vi "PH_Timing.set Attr and open DIM Services.vi"(0 "i ref in":refnum<vi>, 5 "error in (no error)":errorcluster) -> (14 "i ref out":refnum<vi>, 16 "i Attr":T1={"Sequencer"={"linked?"=FALSE, "Proc State"="no info", "Ref State"=refnum}, "Gate Generator"={"GD"={"Device Status"=0, "linked?"=FALSE}, "Settings"={"Instance"="N/A", "Channel Gate"=1, "Channel T2"=1, "Width Gate"=1.0, "Width T2"=1.0, "Delay Gate"=0.0, "Delay T2"=0.0, "Gate activ"=FALSE, "T2 activ"=FALSE, "System Mode"=enum."Normal"}, "GUI Ref"=refnum}, "Interlock Bypass"={"Instancename"="N/A", "Switch linked?"=FALSE, "Device Status"=0, "Ref Status"=refnum}, "Roughtuner"={"Settings"={"Instance"="N/A", "Phase PHELIX / UNILAC"={"Channel"=0, "relative to"=0, "Delay [ms]"=0.0}, "Pulse Length"={"Channel"=0, "relative to"=0, "Delay [ms]"=0.0}, "Trigger"={"externally?"=FALSE, "Rate [Hz]"=0.0}}, "GUI Ref"=refnum, "GD"={"Device Status"=0, "linked?"=FALSE}}, "0,5Hz Gater"={"Settings"={"Instance"="N/A", "Channel ns FE Delay"=1, "Channel 0.5Hz"=1, "Width ns FE Delay"=1.0, "Width 0.5Hz"=1.0, "Delay ns FE Delay"=0.0, "Delay 0.5Hz"=0.0, "ns FE Delay active"=FALSE, "0.5Hz activ"=FALSE, "ns FE Delay inverted"=FALSE, "0.5Hz inverted"=FALSE}, "GUI Ref"=refnum, "GD"={"Device Status"=0, "linked?"=FALSE}}, "Slow Trigger"={"Settings"={"Delay"=0.0, "externally triggered?"=FALSE}, "GUI Ref"=refnum, "Service ID Delay"=-1, "Service ID Ext Trig"=-1, "Wanted Settings"={"Delay"=0.0, "externally triggered?"=FALSE}}, "Timing Mode"={"Mode"={"T2"=0, "Modeselector"=enum."0.5 Hz"}, "GUI Ref"=refnum, "Service ID T2"=-1, "Service ID Mode"=-1, "Wanted Mode"={"T2"=0, "Modeselector"=enum."10 Hz"}}, "ns Generator"={"Settings"={"Instance"="N/A", "Phase fs / ns FE"={"Channel"=0, "Settings"={"Delay [s]"=0.0, "relative to"=0}}}, "ns Generator Settings"=refnum, "GD"={"Device Status"=0, "linked?"=FALSE}}, "Phase FEs"={"Settings"={"Phase"=0.0}, "GUI Ref"=refnum, "Service ID Phase"=-1, "Wanted Settings"={"Phase"=0.0}}, "GD GUI Refs"=[], "Heads"=[], "GUI Ref Delete"=refnum} {"Heads"."GD"."Device Status" items=["no info", "off/false/out", "on/true/in", "Failure", "Alarm", "Status 1", "Status 2", "Status 3"]; "Heads"."Data"."CH" items=["System (To)", "Channel A", "Channel B", "Channel C", "Channel D", "Channel E", "Channel F", "Channel G", "Channel H"]; "Heads"."Data"."Delay" format="%#_7f"; "Phase FEs"."Wanted Settings"."Phase" format="%#_12p"; "Phase FEs"."Settings"."Phase" format="%#_12p"; "ns Generator"."GD"."Device Status" items=["no info", "off/false/out", "on/true/in", "Failure", "Alarm", "Status 1", "Status 2", "Status 3"]; "ns Generator"."Settings"."Phase fs / ns FE"."Settings"."relative to" items=["T0", "T1", "A", "B", "C", "D", "E", "F", "G", "H"]; "ns Generator"."Settings"."Phase fs / ns FE"."Settings"."Delay [s]" format="%#_12p"; "ns Generator"."Settings"."Phase fs / ns FE"."Channel" items=["T0", "T1", "A", "B", "C", "D", "E", "F", "G", "H"]; "Timing Mode"."Wanted Mode"."T2" min=0 max=6000 step=2; "Timing Mode"."Mode"."T2" min=0 max=6000 step=2; "0,5Hz Gater"."GD"."Device Status" items=["no info", "off/false/out", "on/true/in", "Failure", "Alarm", "Status 1", "Status 2", "Status 3"]; "0,5Hz Gater"."Settings"."Channel ns FE Delay" items=["System (To)", "Channel A", "Channel B", "Channel C", "Channel D", "Channel E", "Channel F", "Channel G", "Channel H"]; "0,5Hz Gater"."Settings"."Channel 0.5Hz" items=["System (To)", "Channel A", "Channel B", "Channel C", "Channel D", "Channel E", "Channel F", "Channel G", "Channel H"]; "Roughtuner"."GD"."Device Status" items=["no info", "off/false/out", "on/true/in", "Failure", "Alarm", "Status 1", "Status 2", "Status 3"]; "Roughtuner"."Settings"."Pulse Length"."Delay [ms]" format="%#_8g"; "Roughtuner"."Settings"."Pulse Length"."relative to" items=["T0", "A", "B", "AB", "C", "D", "CD"]; "Roughtuner"."Settings"."Pulse Length"."Channel" items=["T0", "A", "B", "AB", "C", "D", "CD"]; "Roughtuner"."Settings"."Phase PHELIX / UNILAC"."Delay [ms]" format="%#_8g"; "Roughtuner"."Settings"."Phase PHELIX / UNILAC"."relative to" items=["T0", "A", "B", "AB", "C", "D", "CD"]; "Roughtuner"."Settings"."Phase PHELIX / UNILAC"."Channel" items=["T0", "A", "B", "AB", "C", "D", "CD"]; "Interlock Bypass"."Device Status" items=["no info", "off/false/out", "on/true/in", "Failure", "Alarm", "Status 1", "Status 2", "Status 3"]; "Gate Generator"."Settings"."Channel Gate" items=["System (To)", "Channel A", "Channel B", "Channel C", "Channel D", "Channel E", "Channel F", "Channel G", "Channel H"]; "Gate Generator"."Settings"."Channel T2" items=["System (To)", "Channel A", "Channel B", "Channel C", "Channel D", "Channel E", "Channel F", "Channel G", "Channel H"]; "Gate Generator"."GD"."Device Status" items=["no info", "off/false/out", "on/true/in", "Failure", "Alarm", "Status 1", "Status 2", "Status 3"]}, 19 "error out":errorcluster)   [LabVIEW 2014, in "PH_Timing.lvlib"]
doc: "In this VI the related instances which are not set in the Read DB Vi are defined and set (includinbg default values) to own attributes."
uses:
  PH_Timing.lvlib
  PH_Timing.i attribute.ctl
  PH_Basics/PH_StatusHandler/PH_StatusHandler.Status.ctl
  PH_Timing.GateGen.ctl
  PH_Timing.Roughtuner.ctl
  PH_Timing.0.5HzGater.ctl
  PH_Timing.Slow Trigger Settings.ctl
  PH_Timing.Timing Mode.ctl
  PH_Timing.ns Generator.ctl
  instr.lib/SRDG645/Driver/Channel.ctl
  PH_Devices/PH_SRDG645/PH_SRDG645.Channel Settings.ctl
  PH_Timing.Phase FEs.ctl
  PH_Timing.PU Data.ctl
  PH_Timing.PU Info.ctl
  PH_Basics/PH_PP_Common/PH_PP_Common.PUs.ctl
  CS_DigitalIO/SRDG535/SRDG535.Channel.ctl
  CS_DigitalIO/SRDG535/SRDG535.lvlib
  instr.lib/SRDG645/Stanford Research DG645 - Driver.lvlib
  PH_Basics/PH_StatusHandler/PH_StatusHandler.lvlib
  PH_Devices/PH_SRDG645/PH_SRDG645.lvlib
  PH_Basics/PH_Common/PH_Common.lvlib
  PH_Basics/PH_PP_Common/PH_PP_Common.lvlib
  CS_Core/CSSystem/CSSystemLib/CSSystemLib.lvlib
panel:
  # "s"
  # "s"
  # "AND ns FE Delay"
  # "AND 0.5 Hz"
  # "Gate"
  # "T2"
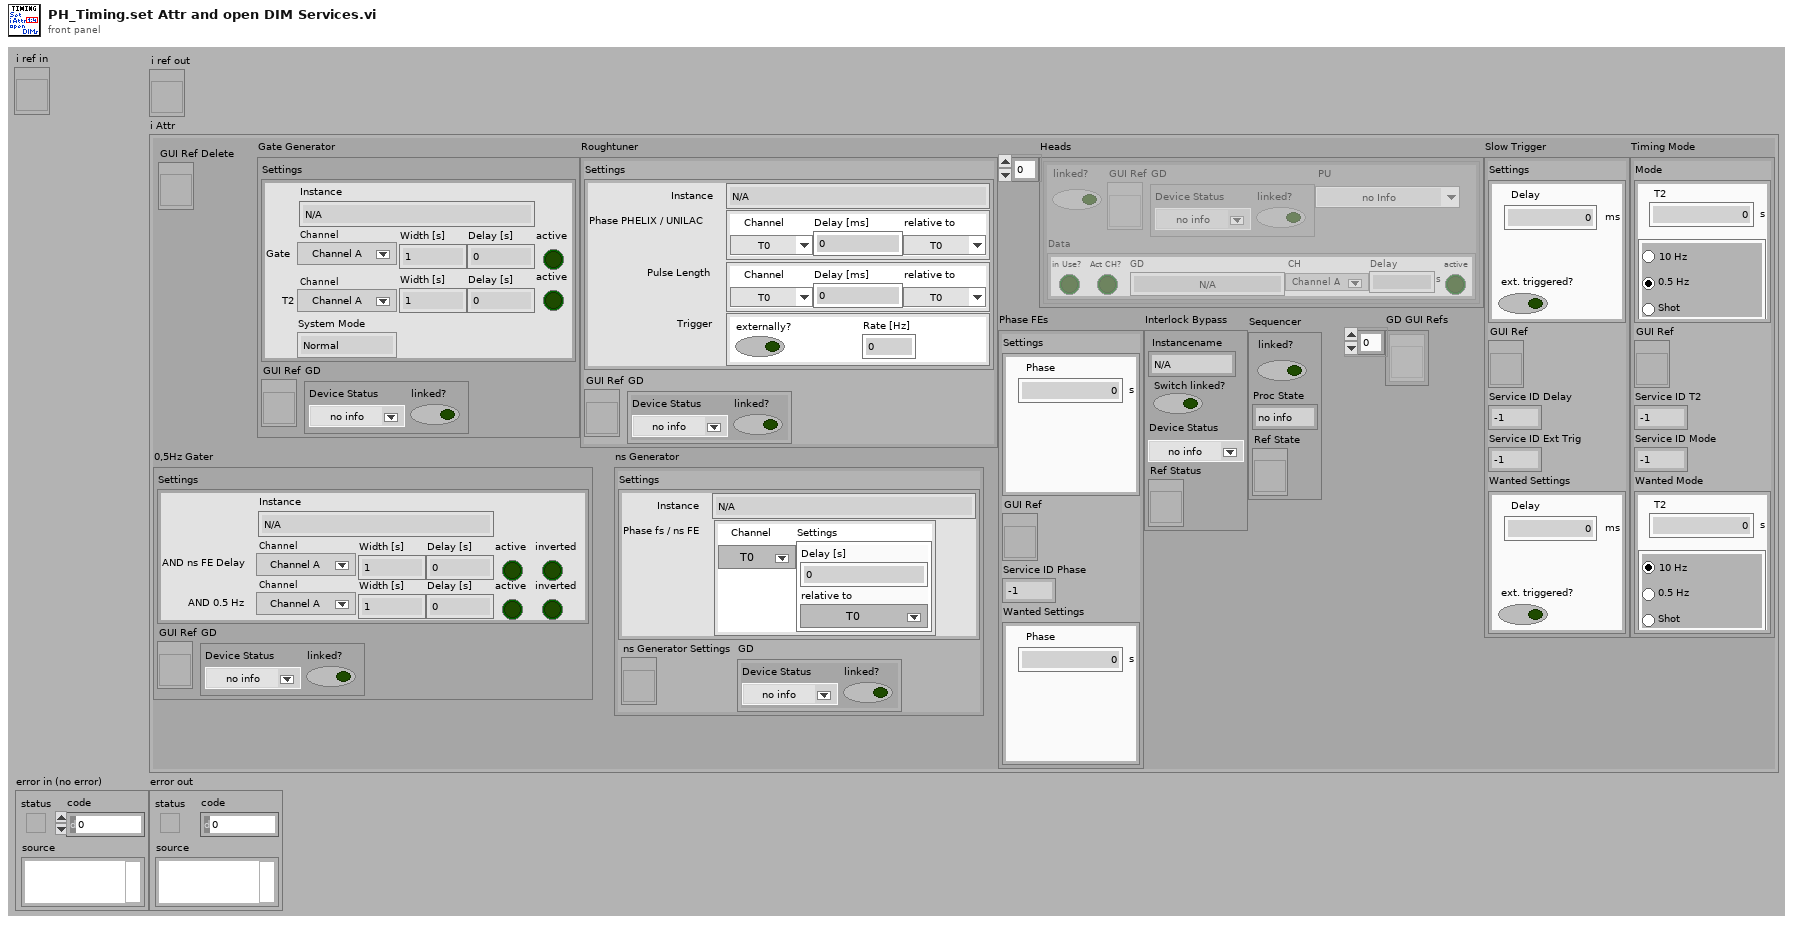
[diagram p1: front panel]
types:
  T1 = typedef "PH_Timing.lvlib/PH_Timing.i attribute.ctl" = cluster{"Sequencer":cluster{"linked?":bool, "Proc State":string, "Ref State":refnum<vi>}, "Gate Generator":cluster{"GD":cluster{"Device Status":T2, "linked?":bool}, "Settings":T3, "GUI Ref":refnum<vi>}, "Interlock Bypass":cluster{"Instancename":string, "Switch linked?":bool, "Device Status":T2, "Ref Status":refnum<vi>}, "Roughtuner":cluster{"Settings":T4, "GUI Ref":refnum<vi>, "GD":cluster{"Device Status":T2, "linked?":bool}}, "0,5Hz Gater":cluster{"Settings":T5, "GUI Ref":refnum<vi>, "GD":cluster{"Device Status":T2, "linked?":bool}}, "Slow Trigger":cluster{"Settings":T6, "GUI Ref":refnum<vi>, "Service ID Delay":i32, "Service ID Ext Trig":i32, "Wanted Settings":T6}, "Timing Mode":cluster{"Mode":T7, "GUI Ref":refnum<vi>, "Service ID T2":i32, "Service ID Mode":i32, "Wanted Mode":T7}, "ns Generator":cluster{"Settings":T8, "ns Generator Settings":refnum<vi>, "GD":cluster{"Device Status":T2, "linked?":bool}}, "Phase FEs":cluster{"Settings":T11, "GUI Ref":refnum<vi>, "Service ID Phase":i32, "Wanted Settings":T11}, "GD GUI Refs":refnum<vi>[], "Heads":T12[], "GUI Ref Delete":refnum<vi>}
  T2 = typedef "PH_StatusHandler.lvlib/PH_StatusHandler.Status.ctl" = i16
  T3 = typedef "PH_Timing.lvlib/PH_Timing.GateGen.ctl" = cluster{"Instance":string, "Channel Gate":i32, "Channel T2":i32, "Width Gate":dbl, "Width T2":dbl, "Delay Gate":dbl, "Delay T2":dbl, "Gate activ":bool, "T2 activ":bool, "System Mode":enum16{"Normal", "Single", "Burst", "Duty Cycle"}}
  T4 = typedef "PH_Timing.lvlib/PH_Timing.Roughtuner.ctl" = cluster{"Instance":string, "Phase PHELIX / UNILAC":cluster{"Channel":u16, "relative to":u16, "Delay [ms]":dbl}, "Pulse Length":cluster{"Channel":u16, "relative to":u16, "Delay [ms]":dbl}, "Trigger":cluster{"externally?":bool, "Rate [Hz]":dbl}}
  T5 = typedef "PH_Timing.lvlib/PH_Timing.0.5HzGater.ctl" = cluster{"Instance":string, "Channel ns FE Delay":i32, "Channel 0.5Hz":i32, "Width ns FE Delay":dbl, "Width 0.5Hz":dbl, "Delay ns FE Delay":dbl, "Delay 0.5Hz":dbl, "ns FE Delay active":bool, "0.5Hz activ":bool, "ns FE Delay inverted":bool, "0.5Hz inverted":bool}
  T6 = typedef "PH_Timing.lvlib/PH_Timing.Slow Trigger Settings.ctl" = cluster{"Delay":dbl, "externally triggered?":bool}
  T7 = typedef "PH_Timing.lvlib/PH_Timing.Timing Mode.ctl" = cluster{"T2":i16, "Modeselector":enum32{"10 Hz", "0.5 Hz", "Shot"}}
  T8 = typedef "PH_Timing.lvlib/PH_Timing.ns Generator.ctl" = cluster{"Instance":string, "Phase fs / ns FE":cluster{"Channel":T9, "Settings":T10}}
  T9 = typedef "Stanford Research DG645 - Driver.lvlib/Channel.ctl" = i32
  T10 = typedef "PH_SRDG645.lvlib/PH_SRDG645.Channel Settings.ctl" = cluster{"Delay [s]":dbl, "relative to":i32}
  T11 = typedef "PH_Timing.lvlib/PH_Timing.Phase FEs.ctl" = cluster{"Phase":dbl}
  T12 = typedef "PH_Timing.lvlib/PH_Timing.PU Data.ctl" = cluster{"linked?":bool, "Data":T13, "GD":cluster{"Device Status":T2, "linked?":bool}, "GUI Ref":refnum<vi>, "PU":T14}
  T13 = typedef "PH_Timing.lvlib/PH_Timing.PU Info.ctl" = cluster{"Act CH?":bool, "GD":string, "CH":i32, "Delay":dbl, "active":bool, "in Use?":bool}
  T14 = typedef "PH_PP_Common.lvlib/PH_PP_Common.PUs.ctl" = enum16{"no Info", "PA-19mm-1", "PA-19mm-2", "PA-45mm-PILC", "PA-45mm-MAIN", "MA-PU-1", "MA-PU-2", "MA-PU-3", "MA-PU-4", "MA-PU-5", "MA-PU-6", "MA-FR", "MA-PILC", "PA-45mm-DP"}
  T15 = typedef "SRDG535.lvlib/SRDG535.Channel.ctl" = u16
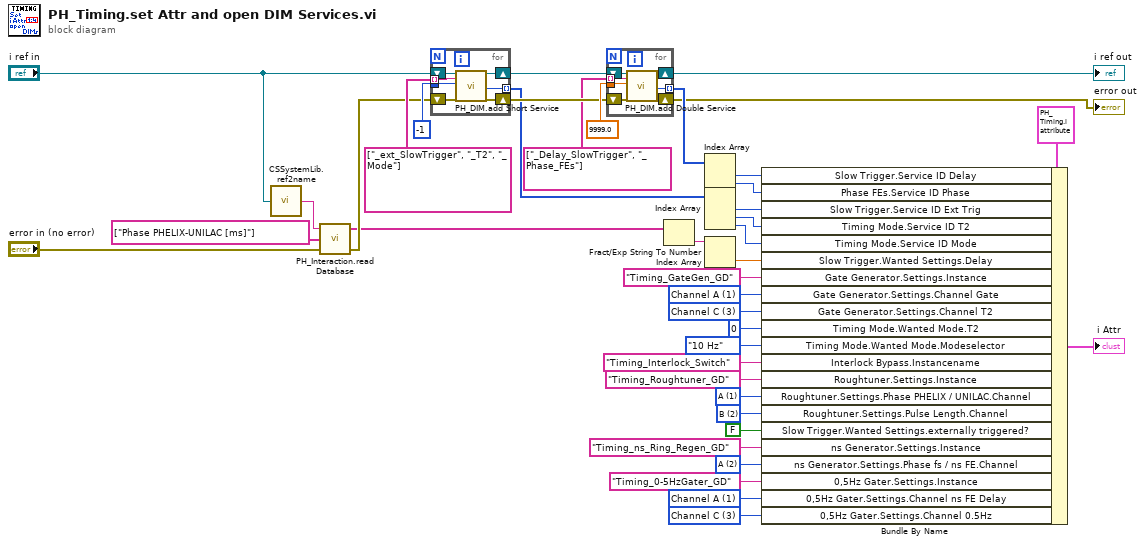
[diagram p0: block diagram]
diagram:
  w15 = T9 2 items=["T0", "T1", "A", "B", "C", "D", "E", "F", "G", "H"] ("ns Generator.Settings.Phase fs / ns FE.Channel")
  w34 = T15 2 items=["T0", "A", "B", "AB", "C", "D", "CD"] ("Channel")
  w35 = T15 1 items=["T0", "A", "B", "AB", "C", "D", "CD"] ("Channel")
  w37 = 3 items=["System (To)", "Channel A", "Channel B", "Channel C", "Channel D", "Channel E", "Channel F", "Channel G", "Channel H"] ("Channel Gate T0")
  w38 = 1 items=["System (To)", "Channel A", "Channel B", "Channel C", "Channel D", "Channel E", "Channel F", "Channel G", "Channel H"] ("Channel Gate T0")
  w39 = 3 items=["System (To)", "Channel A", "Channel B", "Channel C", "Channel D", "Channel E", "Channel F", "Channel G", "Channel H"] ("Channel Gate T0")
  w40 = 1 items=["System (To)", "Channel A", "Channel B", "Channel C", "Channel D", "Channel E", "Channel F", "Channel G", "Channel H"] ("Channel Gate T0")
  n1 = call "CSSystemLib.ref2name.vi"("obj refnum"="i ref in") -> ("name"=w11:string)
  n2 = call "PH_Interaction.read Database.vi"("error in (no error)"="error in (no error)", "Strings to search for"=string[] ["Phase PHELIX-UNILAC [ms]"], "DB Entry to read"=w11) -> ("error out"=w13:errorcluster, "Values"=w12:string[])  [unwired: 1 in]
  n3 = for {
    tunnel: i16 -1 ("Number") -> [w45]
    shift-right: [w47] -> w27
    shift-left: "i ref in" -> [w44]
    shift-right: [w46] -> w26
    shift-left: w13 -> [w43]
    tunnel: string[] ["_ext_SlowTrigger", "_T2", "_Mode"] -> [w42] mode=indexing
    tunnel: [w41] -> w23 mode=indexing
    n4 = call "PH_DIM.add Short Service.vi"("i ref in"=w44, "Service Name"=w42, "Number"=w45, "error in (no error)"=w43) -> ("i ref out"=w47:refnum<vi>, "Service ID"=w41:i32, "error out"=w46:errorcluster)  [unwired: 13 in]
  }
  n5 = for {
    tunnel: 9999.0 ("Double Value") -> [w52]
    tunnel: [w49] -> w21 mode=indexing
    tunnel: string[] ["_Delay_SlowTrigger", "_Phase_FEs"] -> [w48] mode=indexing
    shift-right: [w54] -> w2
    shift-left: w27 -> [w51]
    shift-right: [w53] -> w1
    shift-left: w26 -> [w50]
    n6 = call "PH_DIM.add Double Service.vi"("i ref in"=w51, "Service Name"=w48, "Double Value"=w52, "error in (no error)"=w50) -> ("i ref out"=w54:refnum<vi>, "Service ID"=w49:i32, "error out"=w53:errorcluster)  [unwired: 13 in]
  }
  "error out" <- w1
  "i ref out" <- w2
  n7 = Index Array(array=w12) -> (element=w30:string)  [unwired: 1 in]
  n8 = Index Array(array=w21) -> (element #1=w16:i32, element #2=w17:i32)  [unwired: 2 in]
  n9 = Index Array(array=w23) -> (element #1=w18:i32, element #2=w19:i32, element #3=w20:i32)  [unwired: 3 in]
  n10 = Fract/Exp String To Number(string=w30) -> (number=w29:dbl)  [unwired: 3 in, 1 out]
  n11 = Bundle By Name(cluster=T1 {"Sequencer"={"linked?"=FALSE, "Proc State"="", "Ref State"=refnum}, "Gate Generator"={"GD"={"Device Status"=0, "linked?"=FALSE}, "Settings"={"Instance"="", "Channel Gate"=0, "Channel T2"=0, "Width Gate"=0.0, "Width T2"=0.0, "Delay Gate"=0.0, "Delay T2"=0.0, "Gate activ"=FALSE, "T2 activ"=FALSE, "System Mode"=enum."Normal"}, "GUI Ref"=refnum}, "Interlock Bypass"={"Instancename"="", "Switch linked?"=FALSE, "Device Status"=0, "Ref Status"=refnum}, "Roughtuner"={"Settings"={"Instance"="", "Phase PHELIX / UNILAC"={"Channel"=0, "relative to"=0, "Delay [ms]"=0.0}, "Pulse Length"={"Channel"=0, "relative to"=0, "Delay [ms]"=0.0}, "Trigger"={"externally?"=FALSE, "Rate [Hz]"=0.0}}, "GUI Ref"=refnum, "GD"={"Device Status"=0, "linked?"=FALSE}}, "0,5Hz Gater"={"Settings"={"Instance"="", "Channel ns FE Delay"=0, "Channel 0.5Hz"=0, "Width ns FE Delay"=0.0, "Width 0.5Hz"=0.0, "Delay ns FE Delay"=0.0, "Delay 0.5Hz"=0.0, "ns FE Delay active"=FALSE, "0.5Hz activ"=FALSE, "ns FE Delay inverted"=FALSE, "0.5Hz inverted"=FALSE}, "GUI Ref"=refnum, "GD"={"Device Status"=0, "linked?"=FALSE}}, "Slow Trigger"={"Settings"={"Delay"=0.0, "externally triggered?"=FALSE}, "GUI Ref"=refnum, "Service ID Delay"=0, "Service ID Ext Trig"=0, "Wanted Settings"={"Delay"=0.0, "externally triggered?"=FALSE}}, "Timing Mode"={"Mode"={"T2"=0, "Modeselector"=enum."10 Hz"}, "GUI Ref"=refnum, "Service ID T2"=0, "Service ID Mode"=0, "Wanted Mode"={"T2"=0, "Modeselector"=enum."10 Hz"}}, "ns Generator"={"Settings"={"Instance"="", "Phase fs / ns FE"={"Channel"=0, "Settings"={"Delay [s]"=0.0, "relative to"=0}}}, "ns Generator Settings"=refnum, "GD"={"Device Status"=0, "linked?"=FALSE}}, "Phase FEs"={"Settings"={"Phase"=0.0}, "GUI Ref"=refnum, "Service ID Phase"=0, "Wanted Settings"={"Phase"=0.0}}, "GD GUI Refs"=[], "Heads"=[], "GUI Ref Delete"=refnum} ("i Attr"), "Slow Trigger.Service ID Delay"=w16, "Phase FEs.Service ID Phase"=w17, "Slow Trigger.Service ID Ext Trig"=w18, "Timing Mode.Service ID T2"=w19, "Timing Mode.Service ID Mode"=w20, "Slow Trigger.Wanted Settings.Delay"=w29, "Gate Generator.Settings.Instance"="Timing_GateGen_GD", "Gate Generator.Settings.Channel Gate"=w40, "Gate Generator.Settings.Channel T2"=w39, "Timing Mode.Wanted Mode.T2"=i16 0 ("Timing Mode.Wanted Mode.T2 [s]"), "Timing Mode.Wanted Mode.Modeselector"=enum32{"10 Hz", "0.5 Hz", "Shot"}."10 Hz", "Interlock Bypass.Instancename"="Timing_Interlock_Switch", "Roughtuner.Settings.Instance"="Timing_Roughtuner_GD", "Roughtuner.Settings.Phase PHELIX / UNILAC.Channel"=w35, "Roughtuner.Settings.Pulse Length.Channel"=w34, "Slow Trigger.Wanted Settings.externally triggered?"=FALSE, "ns Generator.Settings.Instance"="Timing_ns_Ring_Regen_GD", "ns Generator.Settings.Phase fs / ns FE.Channel"=w15, "0,5Hz Gater.Settings.Instance"="Timing_0-5HzGater_GD", "0,5Hz Gater.Settings.Channel ns FE Delay"=w38, "0,5Hz Gater.Settings.Channel 0.5Hz"=w37) -> (→"i Attr":T1)
